vi "TCP Queue Ref Holder.vi"(6 "Hold":bool, 8 "error in (no error)":errorcluster, 11 "TCP Queue":refnum<queue>) -> (0 "error out":errorcluster, 3 "Input Queue":refnum<queue>)   [LabVIEW 2014, in "TCP.lvlib"]
uses:
  TCP.lvlib
  support/Message Queue/Message Cluster.ctl
  support/Message Queue/Message Queue.lvlib
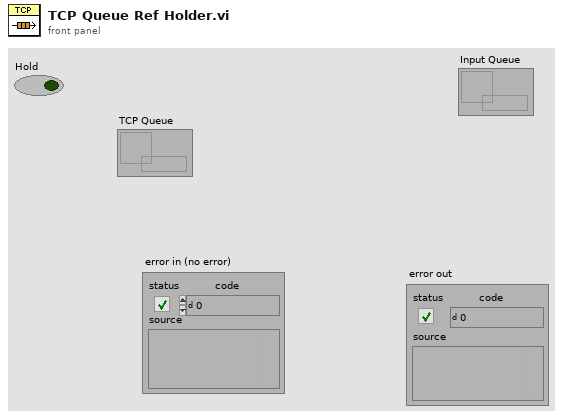
[diagram p1: front panel]
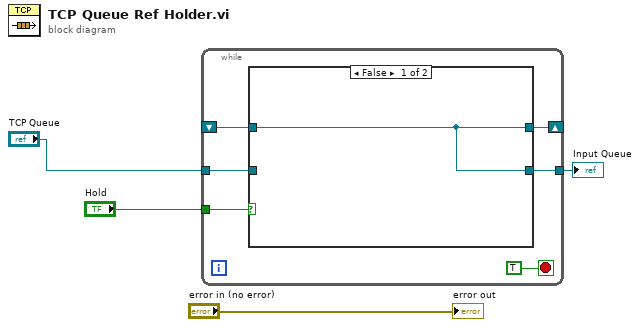
[diagram p0: block diagram]
diagram:
  n1 = while {
    shift-right: [w8] -> _
    shift-left: _ -> [w5]
    tunnel: "TCP Queue" -> [w7]
    tunnel: "Hold" -> [w9]
    tunnel: [w6] -> w1
    stop <- TRUE stop-if-true
    n2 = case shown="False" w9 {
      tunnel: [w11 w12] -> w8
      tunnel: w7 -> [_ w12]
      tunnel: [w11 w12] -> w6
      tunnel: w5 -> [w11 _]
      frame False {
      }
      frame True {
      }
    }
  }
  "Input Queue" <- w1
  "error out" <- "error in (no error)"
